vi "JKISM++ Dummy Module.vi"(7 "Name(\"\" to use uuid)":string="JKISM-Module") -> ()   [LabVIEW 2014, in "JKI State Machine++.lvlib"]
doc: "Template for building JKISM++ Module without User Interface.\n\n<b>Inputs:</b>\n- <b>Name(\"\" to use uuid)</b>: Module Name\n - If Input is \"\", an uuid will be used for module name. The module is marked as stand-alone mode and will not be included in module list.\n - If Input end with '#', the module will worked in worker mode. Modules with the same name will shared the same message queue. Any external message will be processed by one of the modules, depends on who is free.\n - Otherwise, the input string will be used as module name, which should be unique in system. JKISM will go to \"Critical Error\" state if duplicated module name is used in system.\n\n<b>Outputs:</b>\n - N/A"
uses:
  JKI State Machine++.lvlib
panel:
  # "Replace this dummy moudule with your own JKISM+ Module"
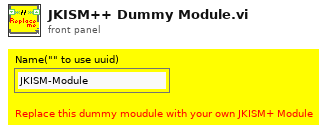
[diagram p1: front panel]
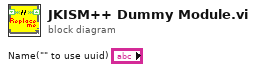
[diagram p0: block diagram]
diagram:
